vi "指令执行.vi"(7 "指令类型":enum16{"standard", "short", "long", "OSD"}(ring), 9 "VISA name":refnum<visa-resource-name>, 10 "COM":bool, 11 "参数数组输入":string[](array[string])) -> (3 "结果输出":string)   [LabVIEW 2016]
uses:
  Global variable.vi
panel:
  in  "vd_cmd_long_header_t":T1
  in  "cmd_short_header_t":T2
  in  "cmd_std_header_t":T3
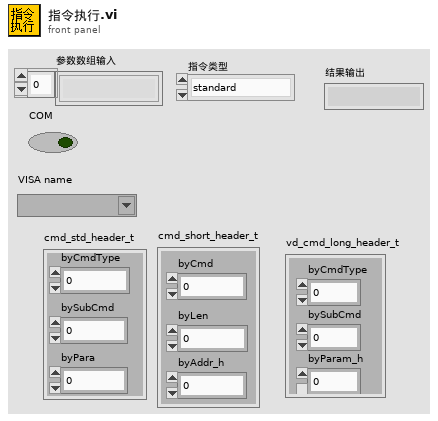
[diagram p1: front panel]
types:
  T1 = cluster{"byCmdType":u8, "bySubCmd":u8, "byParam_h":u8, "byParam_l":u8, "byAddr1_hh":u8, "byAddr1_h":u8, "byAddr1_l":u8, "byAddr1_ll":u8, "byAddr2_hh":u8, "byAddr2_h":u8, "byAddr2_l":u8, "byAddr2_ll":u8, "byLen_hh":u8, "byLen_h":u8, "byLen_l":u8, "byLen_ll":u8}
  T2 = cluster{"byCmd":u8, "byLen":u8, "byAddr_h":u8, "byAddr_l":u8}
  T3 = cluster{"byCmdType":u8, "bySubCmd":u8, "byPara":u8, "byAddr_h":u8, "byAddr_l":u8, "byAddr_ll":u8, "byLen_h":u8, "byLen_l":u8}
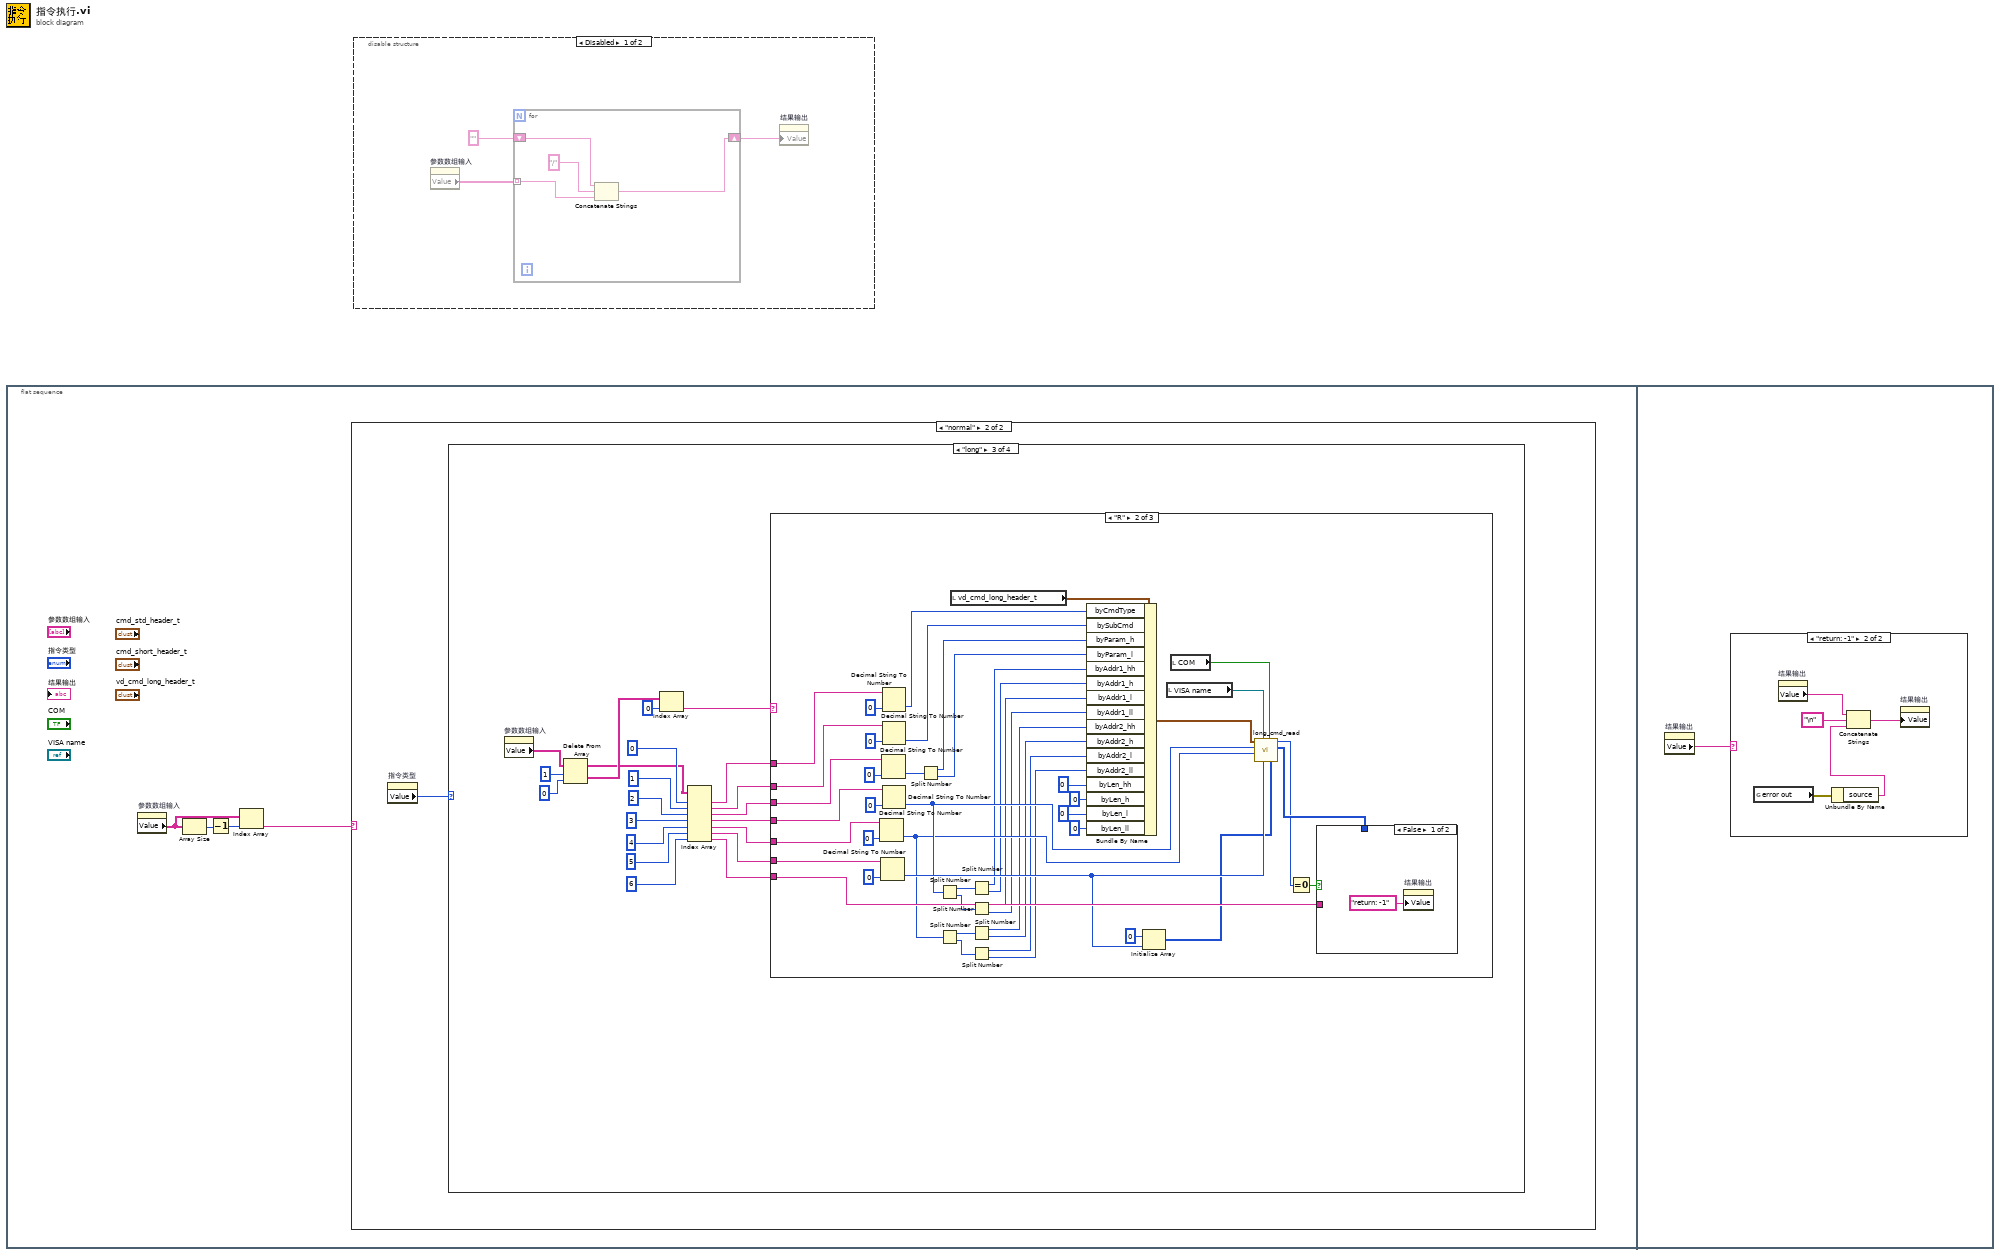
[diagram p0: block diagram]
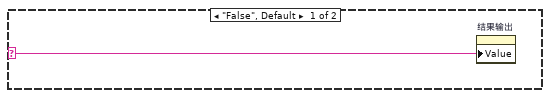
[diagram p2: hidden frame]
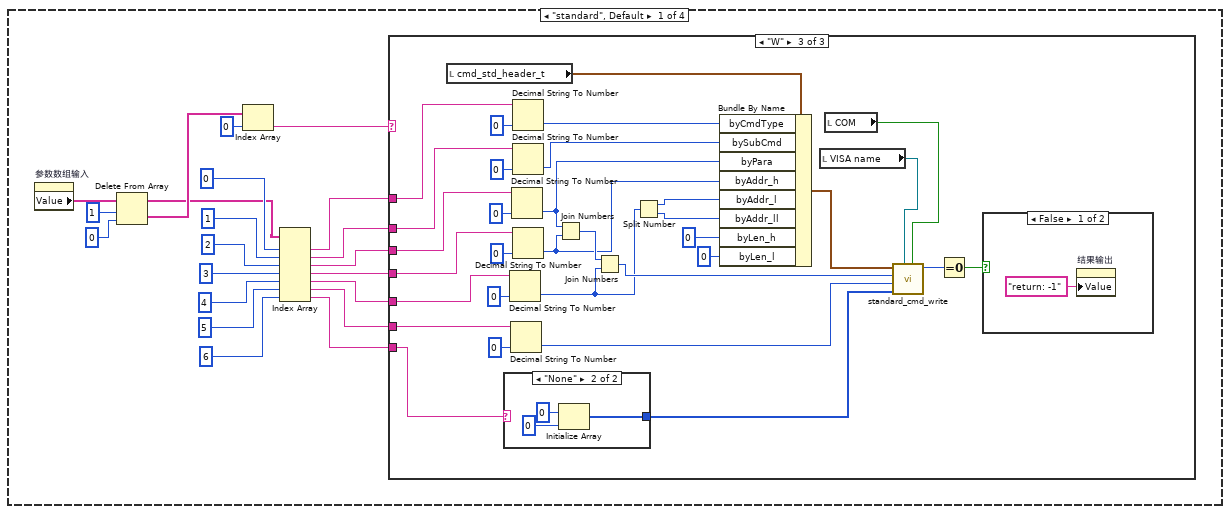
[diagram p3: hidden frame]
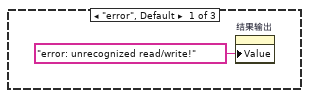
[diagram p4: hidden frame]
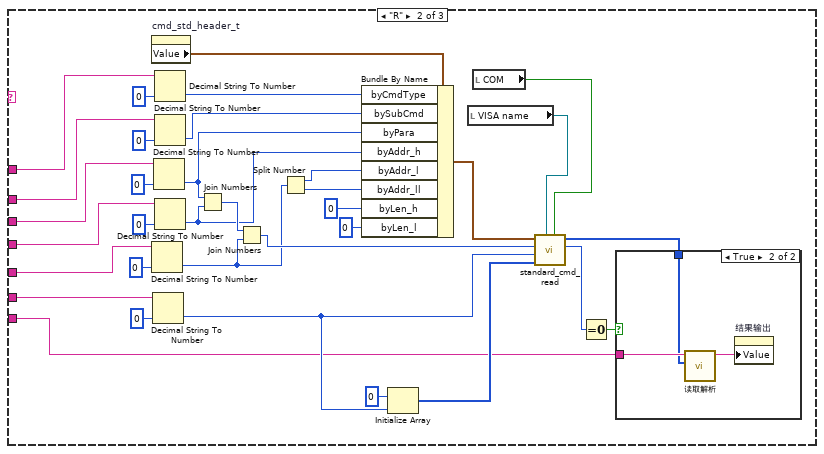
[diagram p5: hidden frame]
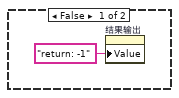
[diagram p6: hidden frame]
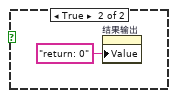
[diagram p7: hidden frame]
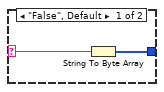
[diagram p8: hidden frame]
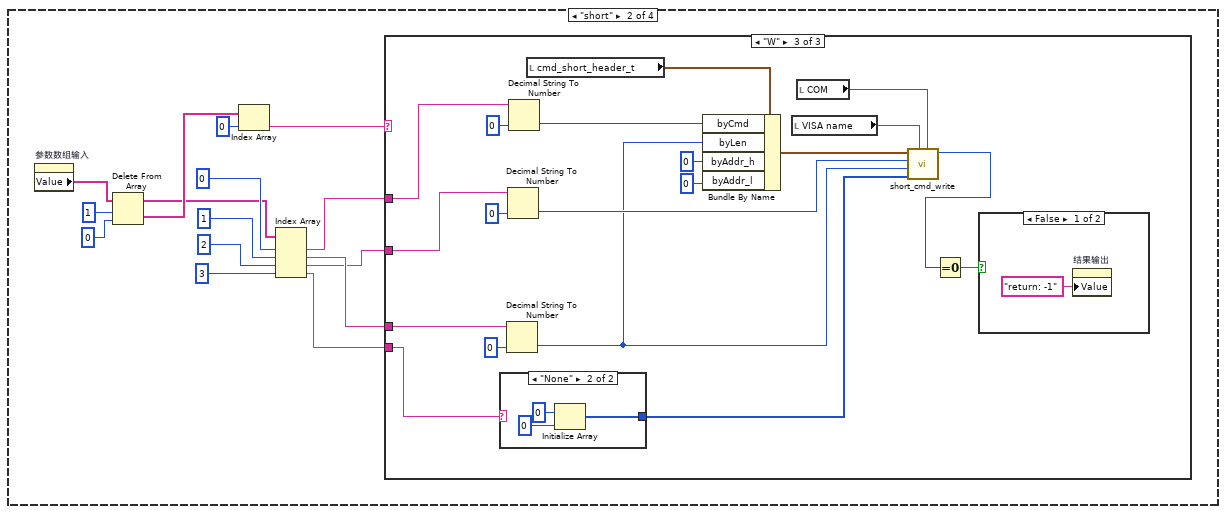
[diagram p9: hidden frame]
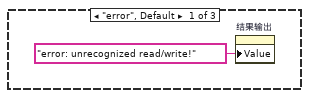
[diagram p10: hidden frame]
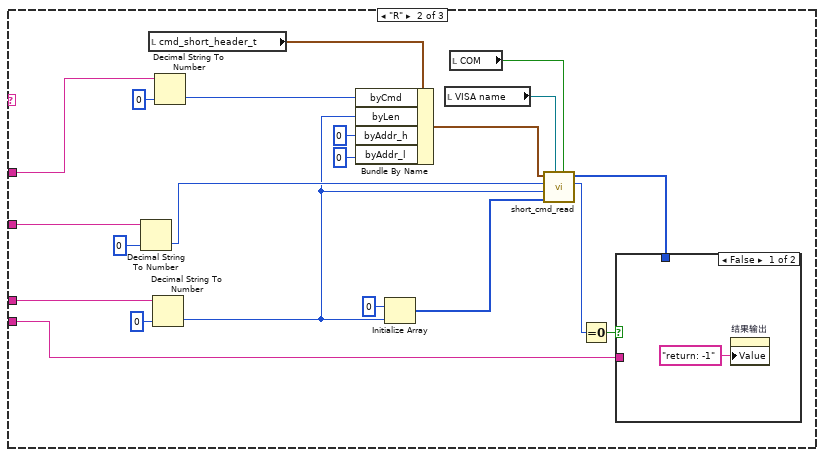
[diagram p11: hidden frame]
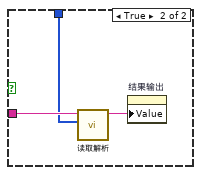
[diagram p12: hidden frame]
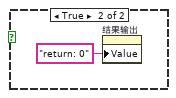
[diagram p13: hidden frame]
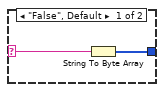
[diagram p14: hidden frame]
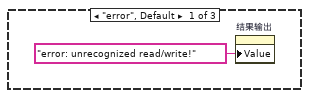
[diagram p15: hidden frame]
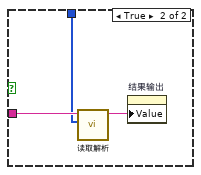
[diagram p16: hidden frame]
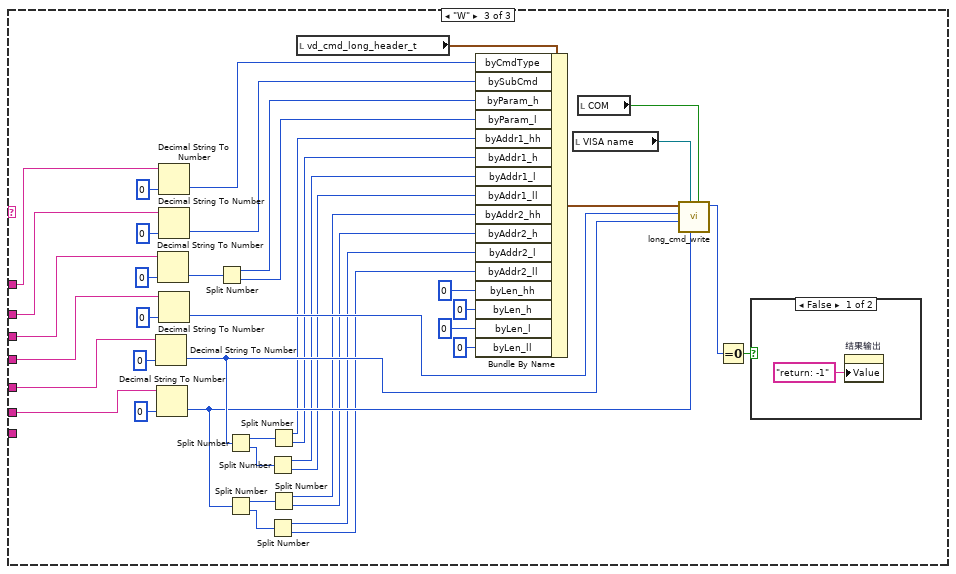
[diagram p17: hidden frame]
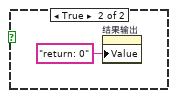
[diagram p18: hidden frame]
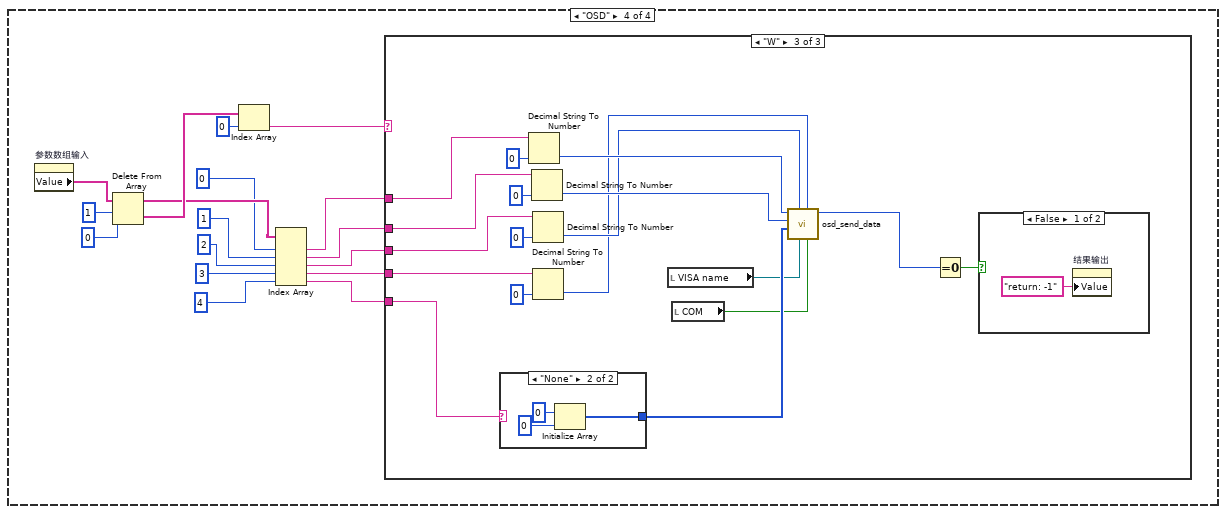
[diagram p19: hidden frame]
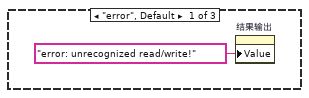
[diagram p20: hidden frame]
diagram:
  n1 = flat-sequence {
    frame #0 {
      n2 = property on="参数数组输入" class="Arr (strict)"() -> ("Value"=w2:string[])  [unwired: 2 in, 2 out]
      n3 = Array Size(array=w2) -> (size(s)=w4:i32)
      n4 = Decrement(x=w4) -> (x-1=w3:i32)
      n5 = Index Array(array=w2, index=w3) -> (element=w1:string)
      n6 = case shown="\"normal\"" w1 {
        selector: w1 -> [w5 _]
        frame "False", Default {
          n7 = property on="结果输出" class="Str"("Value"=w5) -> ()  [unwired: 2 in, 2 out]
        }
        frame "normal" {
          n8 = property on="指令类型" class="Enum (strict)"() -> ("Value"=w6:enum16{"standard", "short", "long", "OSD"})  [unwired: 2 in, 2 out]
          n9 = case shown="\"long\"" w6 {
            frame "standard", Default {
              n10 = property on="参数数组输入" class="Arr (strict)"() -> ("Value"=w27:string[])  [unwired: 2 in, 2 out]
              n11 = Delete From Array(array=w27, length=1, index=0) -> (deleted portion=w17:string[], array with subset deleted=w7:string[])
              n12 = Index Array(array=w17, index=0) -> (element=w15:string)
              n13 = Index Array(array=w7, index #1=0 ("index"), index #2=1 ("index"), index #3=2 ("index"), index #4=3 ("index"), index #5=4 ("index"), index #6=5 ("index"), index #7=6 ("index")) -> (element #1=w14:string, element #2=w13:string, element #3=w12:string, element #4=w11:string, element #5=w10:string, element #6=w9:string, element #7=w8:string)
              n14 = case shown="\"W\"" w15 {
                tunnel: w14 -> [_ w48 w95]
                tunnel: w13 -> [_ w47 w91]
                tunnel: w12 -> [_ w46 w82]
                tunnel: w11 -> [_ w45 w81]
                tunnel: w10 -> [_ w44 w84]
                tunnel: w9 -> [_ w49 w87]
                tunnel: w8 -> [_ w39 w98]
                frame "error", Default {
                  n15 = property on="结果输出" class="Str"("Value"="error: unrecognized read/write!" ("结果输出")) -> ()  [unwired: 2 in, 2 out]
                }
                frame "R" {
                  n16 = property on="cmd_std_header_t" class="Clust (strict)"() -> ("Value"=w40:T3)  [unwired: 2 in, 2 out]
                  n17 = Decimal String To Number(string=w44, default (0L)=u16 0 ("default (0 I32)")) -> (number=w31:u16)  [unwired: 1 in, 1 out]
                  n18 = Decimal String To Number(string=w49, default (0L)=u16 0 ("default (0 I32)")) -> (number=w42:u16)  [unwired: 1 in, 1 out]
                  n19 = Decimal String To Number(string=w46, default (0L)=u8 0 ("default (0 I32)")) -> (number=w33:u8)  [unwired: 1 in, 1 out]
                  n20 = Decimal String To Number(string=w48, default (0L)=u8 0 ("default (0 I32)")) -> (number=w62:u8)  [unwired: 1 in, 1 out]
                  n21 = Decimal String To Number(string=w47, default (0L)=u8 0 ("default (0 I32)")) -> (number=w61:u8)  [unwired: 1 in, 1 out]
                  n22 = Decimal String To Number(string=w45, default (0L)=u8 0 ("default (0 I32)")) -> (number=w32:u8)  [unwired: 1 in, 1 out]
                  n23 = Join Numbers(hi=w33, lo=w32) -> ((hi.lo)=w60:u16)
                  n24 = Join Numbers(hi=w60, lo=w31) -> ((hi.lo)=w59:u32)
                  n25 = Split Number(x=w31) -> (hi(x)=w30:u8, lo(x)=w29:u8)
                  n26 = Bundle By Name(cluster=w40, "byCmdType"=w62, "bySubCmd"=w61, "byPara"=w33, "byAddr_h"=w32, "byAddr_l"=w30, "byAddr_ll"=w29, "byLen_h"=u8 0, "byLen_l"=u8 0) -> (w58:T3)
                  n27 = Initialize Array(u8 0 ("element"), w42) -> (w41:u8[])
                  n28 = local read "VISA name"() -> (w35:refnum<visa-resource-name>)
                  n29 = local read "COM"() -> (w34:bool)
                  n30 = call "standard_cmd_read.vi"("COM"=w34, "VISA name"=w35, "data"=w41, "dwLen"=w42, "dwAddr"=w59, "cmd_std_header_t"=w58) -> ("return"=w37:i32, "data out"=w38:u8[])  [unwired: 4 in]
                  n31 = Equal To 0?(x=w37) -> (x = 0?=w36:bool)
                  n32 = case shown="True" w36 {
                    tunnel: w39 -> [_ w66]
                    tunnel: w38 -> [_ w65]
                    frame False {
                      n33 = property on="结果输出" class="Str"("Value"="return: -1" ("结果输出")) -> ()  [unwired: 2 in, 2 out]
                    }
                    frame True {
                      n34 = call "读取解析.vi"("读取data"=w65, "格式字符串"=w66) -> ("输出字符串"=w64:string)  [unwired: 9 in]
                      n35 = property on="结果输出" class="Str"("Value"=w64) -> ()  [unwired: 2 in, 2 out]
                    }
                  }
                }
                frame "W" {
                  n36 = local read "cmd_std_header_t"() -> (w96:T3)
                  n37 = case shown="\"None\"" w98 {
                    selector: w98 -> [w102 _]
                    tunnel: [w101 w103] -> w97
                    frame "False", Default {
                      n38 = String To Byte Array(string=w102) -> (unsigned byte array=w101:u8[])
                    }
                    frame "None" {
                      n39 = Initialize Array(u8 0 ("element"), 0 ("dimension size")) -> (w103:u8[])
                    }
                  }
                  n40 = Decimal String To Number(string=w84, default (0L)=u16 0 ("default (0 I32)")) -> (number=w68:u16)  [unwired: 1 in, 1 out]
                  n41 = Decimal String To Number(string=w87, default (0L)=u16 0 ("default (0 I32)")) -> (number=w86:u16)  [unwired: 1 in, 1 out]
                  n42 = Decimal String To Number(string=w82, default (0L)=u8 0 ("default (0 I32)")) -> (number=w71:u8)  [unwired: 1 in, 1 out]
                  n43 = Decimal String To Number(string=w95, default (0L)=u8 0 ("default (0 I32)")) -> (number=w93:u8)  [unwired: 1 in, 1 out]
                  n44 = Decimal String To Number(string=w91, default (0L)=u8 0 ("default (0 I32)")) -> (number=w90:u8)  [unwired: 1 in, 1 out]
                  n45 = Decimal String To Number(string=w81, default (0L)=u8 0 ("default (0 I32)")) -> (number=w70:u8)  [unwired: 1 in, 1 out]
                  n46 = Join Numbers(hi=w71, lo=w70) -> ((hi.lo)=w80:u16)
                  n47 = Join Numbers(hi=w80, lo=w68) -> ((hi.lo)=w79:u32)
                  n48 = Split Number(x=w68) -> (hi(x)=w69:u8, lo(x)=w67:u8)
                  n49 = Bundle By Name(cluster=w96, "byCmdType"=w93, "bySubCmd"=w90, "byPara"=w71, "byAddr_h"=w70, "byAddr_l"=w69, "byAddr_ll"=w67, "byLen_h"=u8 0, "byLen_l"=u8 0) -> (w78:T3)
                  n50 = local read "VISA name"() -> (w73:refnum<visa-resource-name>)
                  n51 = local read "COM"() -> (w72:bool)
                  n52 = call "standard_cmd_write.vi"("COM"=w72, "VISA name"=w73, "data"=w97, "dwLen"=w86, "dwAddr"=w79, "cmd_std_header_t"=w78) -> ("return"=w75:i32)  [unwired: 5 in]
                  n53 = Equal To 0?(x=w75) -> (x = 0?=w74:bool)
                  n54 = case shown="False" w74 {
                    frame False {
                      n55 = property on="结果输出" class="Str"("Value"="return: -1" ("结果输出")) -> ()  [unwired: 2 in, 2 out]
                    }
                    frame True {
                      n56 = property on="结果输出" class="Str"("Value"="return: 0" ("结果输出")) -> ()  [unwired: 2 in, 2 out]
                    }
                  }
                }
              }
            }
            frame "short" {
              n57 = property on="参数数组输入" class="Arr (strict)"() -> ("Value"=w120:string[])  [unwired: 2 in, 2 out]
              n58 = Delete From Array(array=w120, length=1, index=0) -> (deleted portion=w113:string[], array with subset deleted=w110:string[])
              n59 = Index Array(array=w113, index=0) -> (element=w111:string)
              n60 = Index Array(array=w110, index #1=0 ("index"), index #2=1 ("index"), index #3=2 ("index"), index #4=3 ("index")) -> (element #1=w107:string, element #2=w108:string, element #3=w106:string, element #4=w109:string)
              n61 = case shown="\"W\"" w111 {
                tunnel: w107 -> [_ w138 w164]
                tunnel: w106 -> [_ w129 w159]
                tunnel: w108 -> [_ w139 w160]
                tunnel: w109 -> [_ w136 w165]
                frame "error", Default {
                  n62 = property on="结果输出" class="Str"("Value"="error: unrecognized read/write!" ("结果输出")) -> ()  [unwired: 2 in, 2 out]
                }
                frame "R" {
                  n63 = Decimal String To Number(string=w129, default (0L)=u16 0 ("default (0 I32)")) -> (number=w128:u16)  [unwired: 1 in, 1 out]
                  n64 = local read "cmd_short_header_t"() -> (w134:T2)
                  n65 = Decimal String To Number(string=w139, default (0L)=u16 0 ("default (0 I32)")) -> (number=w122:u16)  [unwired: 1 in, 1 out]
                  n66 = Decimal String To Number(string=w138, default (0L)=u8 0 ("default (0 I32)")) -> (number=w133:u8)  [unwired: 1 in, 1 out]
                  n67 = Bundle By Name(cluster=w134, "byCmd"=w133, "byLen"=w122, "byAddr_h"=u8 0, "byAddr_l"=u8 0) -> (w132:T2)
                  n68 = Initialize Array(u8 0 ("element"), w122) -> (w127:u8[])
                  n69 = local read "VISA name"() -> (w124:refnum<visa-resource-name>)
                  n70 = local read "COM"() -> (w123:bool)
                  n71 = call "short_cmd_read.vi"("COM"=w123, "VISA name"=w124, "data"=w127, "dwLen"=w122, "dwAddr"=w128, "cmd_short_header_t"=w132) -> ("return"=w125:i32, "data out"=w126:u8[])  [unwired: 4 in]
                  n72 = Equal To 0?(x=w125) -> (x = 0?=w135:bool)
                  n73 = case shown="False" w135 {
                    tunnel: w136 -> [_ w146]
                    tunnel: w126 -> [_ w145]
                    frame False {
                      n74 = property on="结果输出" class="Str"("Value"="return: -1" ("结果输出")) -> ()  [unwired: 2 in, 2 out]
                    }
                    frame True {
                      n75 = call "读取解析.vi"("读取data"=w145, "格式字符串"=w146) -> ("输出字符串"=w144:string)  [unwired: 9 in]
                      n76 = property on="结果输出" class="Str"("Value"=w144) -> ()  [unwired: 2 in, 2 out]
                    }
                  }
                }
                frame "W" {
                  n77 = case shown="\"None\"" w165 {
                    selector: w165 -> [w169 _]
                    tunnel: [w168 w170] -> w152
                    frame "False", Default {
                      n78 = String To Byte Array(string=w169) -> (unsigned byte array=w168:u8[])
                    }
                    frame "None" {
                      n79 = Initialize Array(u8 0 ("element"), 0 ("dimension size")) -> (w170:u8[])
                    }
                  }
                  n80 = Decimal String To Number(string=w160, default (0L)=u16 0 ("default (0 I32)")) -> (number=w147:u16)  [unwired: 1 in, 1 out]
                  n81 = Decimal String To Number(string=w159, default (0L)=u16 0 ("default (0 I32)")) -> (number=w151:u16)  [unwired: 1 in, 1 out]
                  n82 = Decimal String To Number(string=w164, default (0L)=u8 0 ("default (0 I32)")) -> (number=w154:u8)  [unwired: 1 in, 1 out]
                  n83 = local read "cmd_short_header_t"() -> (w157:T2)
                  n84 = Bundle By Name(cluster=w157, "byCmd"=w154, "byLen"=w147, "byAddr_h"=u8 0, "byAddr_l"=u8 0) -> (w153:T2)
                  n85 = local read "VISA name"() -> (w149:refnum<visa-resource-name>)
                  n86 = local read "COM"() -> (w148:bool)
                  n87 = call "short_cmd_write.vi"("COM"=w148, "VISA name"=w149, "data"=w152, "dwLen"=w147, "dwAddr"=w151, "cmd_short_header_t"=w153) -> ("return"=w150:i32)  [unwired: 5 in]
                  n88 = Equal To 0?(x=w150) -> (x = 0?=w158:bool)
                  n89 = case shown="False" w158 {
                    frame False {
                      n90 = property on="结果输出" class="Str"("Value"="return: -1" ("结果输出")) -> ()  [unwired: 2 in, 2 out]
                    }
                    frame True {
                      n91 = property on="结果输出" class="Str"("Value"="return: 0" ("结果输出")) -> ()  [unwired: 2 in, 2 out]
                    }
                  }
                }
              }
            }
            frame "long" {
              n92 = property on="参数数组输入" class="Arr (strict)"() -> ("Value"=w193:string[])  [unwired: 2 in, 2 out]
              n93 = Delete From Array(array=w193, length=1, index=0) -> (deleted portion=w183:string[], array with subset deleted=w173:string[])
              n94 = Index Array(array=w183, index=0) -> (element=w181:string)
              n95 = Index Array(array=w173, index #1=0 ("index"), index #2=1 ("index"), index #3=2 ("index"), index #4=3 ("index"), index #5=4 ("index"), index #6=5 ("index"), index #7=6 ("index")) -> (element #1=w180:string, element #2=w179:string, element #3=w178:string, element #4=w177:string, element #5=w176:string, element #6=w175:string, element #7=w174:string)
              n96 = case shown="\"R\"" w181 {
                tunnel: w180 -> [_ w233 w268]
                tunnel: w179 -> [_ w232 w267]
                tunnel: w178 -> [_ w231 w266]
                tunnel: w177 -> [_ w230 w265]
                tunnel: w176 -> [_ w229 w264]
                tunnel: w175 -> [_ w234 w262]
                tunnel: w174 -> [_ w227 _]
                frame "error", Default {
                  n97 = property on="结果输出" class="Str"("Value"="error: unrecognized read/write!" ("结果输出")) -> ()  [unwired: 2 in, 2 out]
                }
                frame "R" {
                  n98 = Decimal String To Number(string=w229, default (0L)=u32 0 ("default (0 I32)")) -> (number=w203:u32)  [unwired: 1 in, 1 out]
                  n99 = Decimal String To Number(string=w234, default (0L)=u32 0 ("default (0 I32)")) -> (number=w218:u32)  [unwired: 1 in, 1 out]
                  n100 = Decimal String To Number(string=w231, default (0L)=u16 0 ("default (0 I32)")) -> (number=w222:u16)  [unwired: 1 in, 1 out]
                  n101 = Decimal String To Number(string=w233, default (0L)=u8 0 ("default (0 I32)")) -> (number=w224:u8)  [unwired: 1 in, 1 out]
                  n102 = Decimal String To Number(string=w232, default (0L)=u8 0 ("default (0 I32)")) -> (number=w223:u8)  [unwired: 1 in, 1 out]
                  n103 = Decimal String To Number(string=w230, default (0L)=u32 0 ("default (0 I32)")) -> (number=w204:u32)  [unwired: 1 in, 1 out]
                  n104 = Split Number(x=w222) -> (hi(x)=w221:u8, lo(x)=w220:u8)
                  n105 = Split Number(x=w204) -> (hi(x)=w208:u16, lo(x)=w207:u16)
                  n106 = Split Number(x=w203) -> (hi(x)=w205:u16, lo(x)=w206:u16)
                  n107 = local read "vd_cmd_long_header_t"() -> (w225:T1)
                  n108 = Split Number(x=w207) -> (hi(x)=w200:u8, lo(x)=w199:u8)
                  n109 = Split Number(x=w206) -> (hi(x)=w196:u8, lo(x)=w195:u8)
                  n110 = Split Number(x=w208) -> (hi(x)=w202:u8, lo(x)=w201:u8)
                  n111 = Split Number(x=w205) -> (hi(x)=w198:u8, lo(x)=w197:u8)
                  n112 = Bundle By Name(cluster=w225, "byCmdType"=w224, "bySubCmd"=w223, "byParam_h"=w221, "byParam_l"=w220, "byAddr1_hh"=w202, "byAddr1_h"=w201, "byAddr1_l"=w200, "byAddr1_ll"=w199, "byAddr2_hh"=w198, "byAddr2_h"=w197, "byAddr2_l"=w196, "byAddr2_ll"=w195, "byLen_hh"=u8 0, "byLen_h"=u8 0, "byLen_l"=u8 0, "byLen_ll"=u8 0) -> (w219:T1)
                  n113 = Initialize Array(u8 0 ("element"), w218) -> (w217:u8[])
                  n114 = local read "VISA name"() -> (w210:refnum<visa-resource-name>)
                  n115 = local read "COM"() -> (w209:bool)
                  n116 = call "long_cmd_read.vi"("data"=w217, "COM"=w209, "dwLen"=w218, "VISA name"=w210, "dwAddr2"=w203, "dwAddr1"=w204, "vd_cmd_long_header_t"=w219) -> ("data out"=w216:u8[], "return"=w215:i32)  [unwired: 2 in, 1 out]
                  n117 = Equal To 0?(x=w215) -> (x = 0?=w226:bool)
                  n118 = case shown="False" w226 {
                    tunnel: w227 -> [_ w244]
                    tunnel: w216 -> [_ w243]
                    frame False {
                      n119 = property on="结果输出" class="Str"("Value"="return: -1" ("结果输出")) -> ()  [unwired: 2 in, 2 out]
                    }
                    frame True {
                      n120 = call "读取解析.vi"("读取data"=w243, "格式字符串"=w244) -> ("输出字符串"=w242:string)  [unwired: 9 in]
                      n121 = property on="结果输出" class="Str"("Value"=w242) -> ()  [unwired: 2 in, 2 out]
                    }
                  }
                }
                frame "W" {
                  n122 = Decimal String To Number(string=w264, default (0L)=u32 0 ("default (0 I32)")) -> (number=w254:u32)  [unwired: 1 in, 1 out]
                  n123 = Decimal String To Number(string=w262, default (0L)=u32 0 ("default (0 I32)")) -> (number=w253:u32)  [unwired: 1 in, 1 out]
                  n124 = Decimal String To Number(string=w266, default (0L)=u16 0 ("default (0 I32)")) -> (number=w282:u16)  [unwired: 1 in, 1 out]
                  n125 = Decimal String To Number(string=w268, default (0L)=u8 0 ("default (0 I32)")) -> (number=w284:u8)  [unwired: 1 in, 1 out]
                  n126 = Decimal String To Number(string=w267, default (0L)=u8 0 ("default (0 I32)")) -> (number=w283:u8)  [unwired: 1 in, 1 out]
                  n127 = Decimal String To Number(string=w265, default (0L)=u32 0 ("default (0 I32)")) -> (number=w263:u32)  [unwired: 1 in, 1 out]
                  n128 = Split Number(x=w282) -> (hi(x)=w281:u8, lo(x)=w280:u8)
                  n129 = Split Number(x=w254) -> (hi(x)=w258:u16, lo(x)=w257:u16)
                  n130 = Split Number(x=w253) -> (hi(x)=w255:u16, lo(x)=w256:u16)
                  n131 = Split Number(x=w257) -> (hi(x)=w250:u8, lo(x)=w249:u8)
                  n132 = Split Number(x=w256) -> (hi(x)=w246:u8, lo(x)=w245:u8)
                  n133 = Split Number(x=w258) -> (hi(x)=w252:u8, lo(x)=w251:u8)
                  n134 = Split Number(x=w255) -> (hi(x)=w248:u8, lo(x)=w247:u8)
                  n135 = local read "vd_cmd_long_header_t"() -> (w285:T1)
                  n136 = Bundle By Name(cluster=w285, "byCmdType"=w284, "bySubCmd"=w283, "byParam_h"=w281, "byParam_l"=w280, "byAddr1_hh"=w252, "byAddr1_h"=w251, "byAddr1_l"=w250, "byAddr1_ll"=w249, "byAddr2_hh"=w248, "byAddr2_h"=w247, "byAddr2_l"=w246, "byAddr2_ll"=w245, "byLen_hh"=u8 0, "byLen_h"=u8 0, "byLen_l"=u8 0, "byLen_ll"=u8 0) -> (w269:T1)
                  n137 = local read "VISA name"() -> (w260:refnum<visa-resource-name>)
                  n138 = local read "COM"() -> (w259:bool)
                  n139 = call "long_cmd_write.vi"("COM"=w259, "dwLen"=w253, "VISA name"=w260, "dwAddr2"=w254, "dwAddr1"=w263, "vd_cmd_long_header_t"=w269) -> ("return"=w261:i32)  [unwired: 4 in, 1 out]
                  n140 = Equal To 0?(x=w261) -> (x = 0?=w286:bool)
                  n141 = case shown="False" w286 {
                    frame False {
                      n142 = property on="结果输出" class="Str"("Value"="return: -1" ("结果输出")) -> ()  [unwired: 2 in, 2 out]
                    }
                    frame True {
                      n143 = property on="结果输出" class="Str"("Value"="return: 0" ("结果输出")) -> ()  [unwired: 2 in, 2 out]
                    }
                  }
                }
              }
            }
            frame "OSD" {
              n144 = property on="参数数组输入" class="Arr (strict)"() -> ("Value"=w305:string[])  [unwired: 2 in, 2 out]
              n145 = Delete From Array(array=w305, length=1, index=0) -> (deleted portion=w304:string[], array with subset deleted=w297:string[])
              n146 = Index Array(array=w304, index=0) -> (element=w303:string)
              n147 = Index Array(array=w297, index #1=0 ("index"), index #2=1 ("index"), index #3=2 ("index"), index #4=3 ("index"), index #5=4 ("index")) -> (element #1=w302:string, element #2=w301:string, element #3=w300:string, element #4=w299:string, element #5=w298:string)
              n148 = case shown="\"W\"" w303 {
                tunnel: w302 -> [_ w323 w341]
                tunnel: w301 -> [_ w319 w340]
                tunnel: w300 -> [_ w318 w339]
                tunnel: w299 -> [_ w316 w338]
                tunnel: w298 -> [_ w309 w337]
                frame "error", Default {
                  n149 = property on="结果输出" class="Str"("Value"="error: unrecognized read/write!" ("结果输出")) -> ()  [unwired: 2 in, 2 out]
                }
                frame "R" {
                  n150 = Decimal String To Number(string=w323, default (0L)=u8 0 ("default (0 I32)")) -> (number=w315:u8)  [unwired: 1 in, 1 out]
                  n151 = Decimal String To Number(string=w319, default (0L)=u8 0 ("default (0 I32)")) -> (number=w314:u8)  [unwired: 1 in, 1 out]
                  n152 = Decimal String To Number(string=w318, default (0L)=u8 0 ("default (0 I32)")) -> (number=w313:u8)  [unwired: 1 in, 1 out]
                  n153 = Decimal String To Number(string=w316, default (0L)=u8 0 ("default (0 I32)")) -> (number=w312:u8)  [unwired: 1 in, 1 out]
                  n154 = local read "VISA name"() -> (w308:refnum<visa-resource-name>)
                  n155 = local read "COM"() -> (w307:bool)
                  n156 = call "osd_get_data.vi"("bypara"=w312, "COM"=w307, "byIndex"=w313, "VISA name"=w308, "bySubcmd"=w314, "byCmd"=w315) -> ("data out"=w311:u8[], "return"=w310:i32)  [unwired: 4 in]
                  n157 = Equal To 0?(x=w310) -> (x = 0?=w324:bool)
                  n158 = case shown="False" w324 {
                    tunnel: w309 -> [_ w328]
                    tunnel: w311 -> [_ w327]
                    frame False {
                      n159 = property on="结果输出" class="Str"("Value"="return: -1" ("结果输出")) -> ()  [unwired: 2 in, 2 out]
                    }
                    frame True {
                      n160 = call "读取解析.vi"("读取data"=w327, "格式字符串"=w328) -> ("输出字符串"=w326:string)  [unwired: 9 in]
                      n161 = property on="结果输出" class="Str"("Value"=w326) -> ()  [unwired: 2 in, 2 out]
                    }
                  }
                }
                frame "W" {
                  n162 = case shown="\"None\"" w337 {
                    selector: w337 -> [w350 _]
                    tunnel: [w349 w351] -> w345
                    frame "False", Default {
                      n163 = String To Byte Array(string=w350) -> (unsigned byte array=w349:u8[])
                    }
                    frame "None" {
                      n164 = Initialize Array(u8 0 ("element"), 0 ("dimension size")) -> (w351:u8[])
                    }
                  }
                  n165 = Decimal String To Number(string=w341, default (0L)=u8 0 ("default (0 I32)")) -> (number=w336:u8)  [unwired: 1 in, 1 out]
                  n166 = Decimal String To Number(string=w340, default (0L)=u8 0 ("default (0 I32)")) -> (number=w335:u8)  [unwired: 1 in, 1 out]
                  n167 = Decimal String To Number(string=w339, default (0L)=u8 0 ("default (0 I32)")) -> (number=w334:u8)  [unwired: 1 in, 1 out]
                  n168 = Decimal String To Number(string=w338, default (0L)=u8 0 ("default (0 I32)")) -> (number=w333:u8)  [unwired: 1 in, 1 out]
                  n169 = local read "VISA name"() -> (w330:refnum<visa-resource-name>)
                  n170 = local read "COM"() -> (w329:bool)
                  n171 = call "osd_send_data.vi"("COM"=w329, "bypara"=w333, "VISA name"=w330, "byIndex"=w334, "pbyData"=w345, "bySubcmd"=w335, "byCmd"=w336) -> ("return"=w331:i32)  [unwired: 4 in]
                  n172 = Equal To 0?(x=w331) -> (x = 0?=w346:bool)
                  n173 = case shown="False" w346 {
                    frame False {
                      n174 = property on="结果输出" class="Str"("Value"="return: -1" ("结果输出")) -> ()  [unwired: 2 in, 2 out]
                    }
                    frame True {
                      n175 = property on="结果输出" class="Str"("Value"="return: 0" ("结果输出")) -> ()  [unwired: 2 in, 2 out]
                    }
                  }
                }
              }
            }
          }
        }
      }
    }
    frame #1 {
      n176 = property on="结果输出" class="Str"() -> ("Value"=w354:string)  [unwired: 2 in, 2 out]
      n177 = case shown="\"return: -1\"" w354 {
        frame "return: 0", Default {
        }
        frame "return: -1" {
          n178 = global read "Global variable.vi" "error out"() -> (w357:errorcluster)
          n179 = property on="结果输出" class="Str"() -> ("Value"=w359:string)  [unwired: 2 in, 2 out]
          n180 = Unbundle By Name(w357) -> ("source"=w356:string)
          n181 = Concatenate Strings(w359, "\n" ("string"), w356) -> (w355:string)
          n182 = property on="结果输出" class="Str"("Value"=w355) -> ()  [unwired: 2 in, 2 out]
        }
      }
    }
  }
  n183 = disable-structure shown="Disabled" {
    frame Disabled {
      n184 = property on="参数数组输入" class="Arr (strict)"() -> ("Value"=w362:string[])  [unwired: 2 in, 2 out]
      n185 = for {
        tunnel: w362 -> [w364] mode=indexing
        shift-right: [w363] -> w360
        shift-left: "" -> [w366]
        n186 = Concatenate Strings(w366, "/" ("字符串"), w364) -> (w363:string)
      }
      n187 = property on="结果输出" class="Str"("Value"=w360) -> ()  [unwired: 2 in, 2 out]
    }
    frame Enabled {
    }
  }
